vi "TorreHanoi.vi"() -> ()   [LabVIEW 2020]
uses:
  <vilib>/Utility/miscctls.llb/LVPositionTypeDef.ctl
  <vilib>/Utility/miscctls.llb/LVBoundsTypeDef.ctl
panel:
  out "String 2":string
  in  "Instrucciones":bool
  out "array1":dbl[](array[numeric])
  out "Position:Left":i32
  out "array3":dbl[](array[numeric])
  out "array2":dbl[](array[numeric])
  out "Initial position":T1
  out "CtlRef":refnum<vi>
  out "Disco4":bool caption="Disco 1"
  out "Disco3":bool caption="Disco 1"
  out "Disco5":bool caption="Disco 1"
  out "Disco2":bool caption="Disco 1"
  in  "Número de discos":u16(ring) items=["3"=3, "4"=4, "5"=5]
  out "Disco1":bool caption="Disco 1"
  out "Número de movimientos realizados":dbl
  out "Minimo de movimientos":dbl
  out "Boolean":bool
  out "Boolean 2":bool
  out "Boolean 3":bool
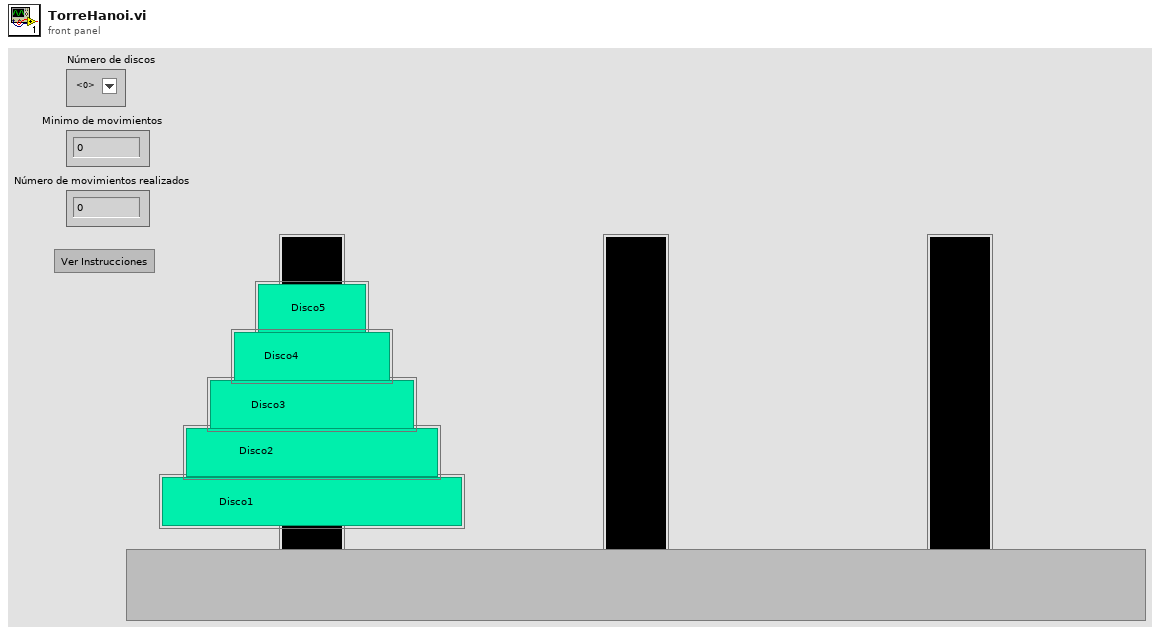
[diagram p1: front panel]
types:
  T1 = typedef "LVPositionTypeDef.ctl" = cluster{"Left":i32, "Top":i32}
  T2 = typedef "LVBoundsTypeDef.ctl" = cluster{"Width":u32, "Height":u32}
  T3 = typedef "LVPoint32TypeDef.ctl" = cluster{"Horizontal":i32, "Vertical":i32}
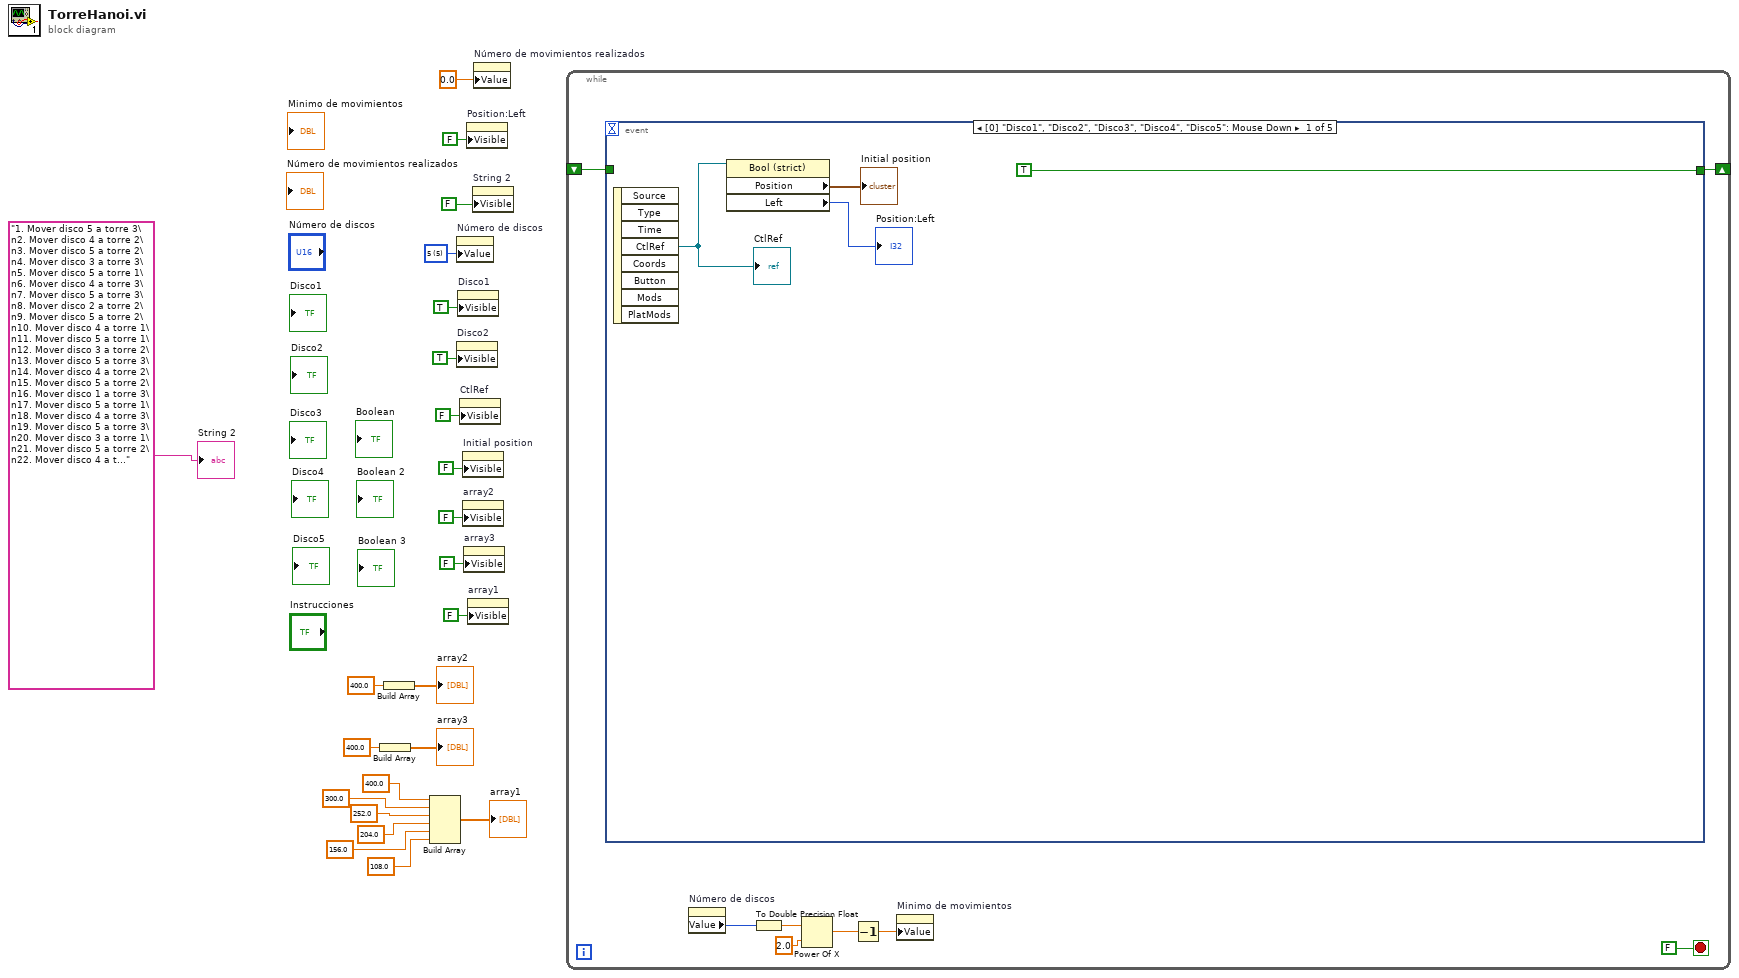
[diagram p0: block diagram]
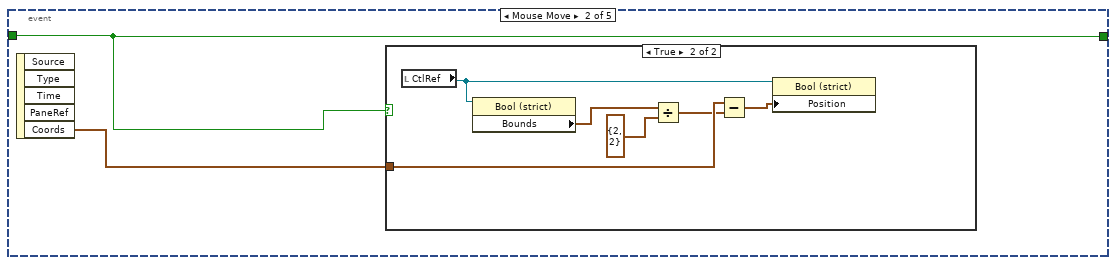
[diagram p2: hidden frame]
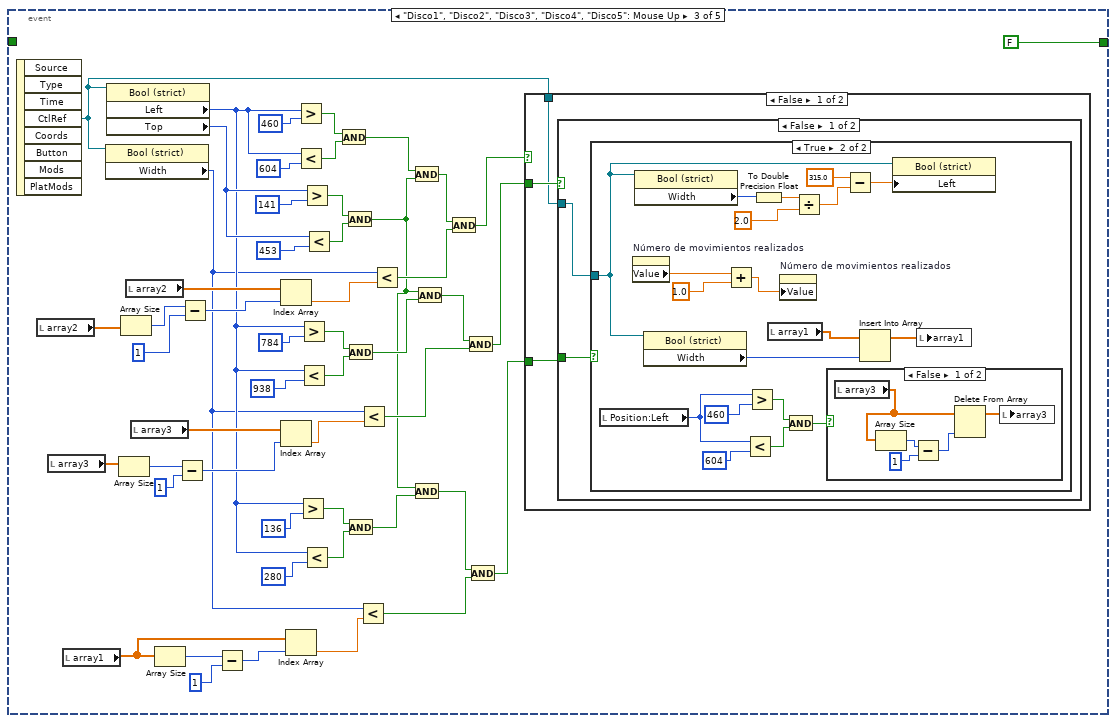
[diagram p4: hidden frame]
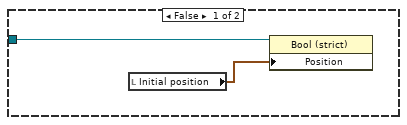
[diagram p5: hidden frame]
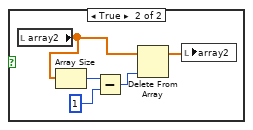
[diagram p6: hidden frame]
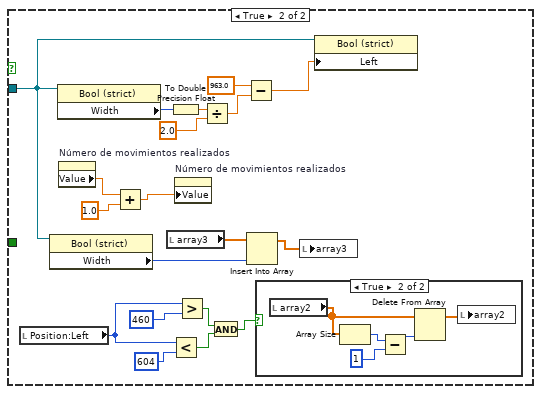
[diagram p7: hidden frame]
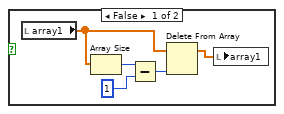
[diagram p8: hidden frame]
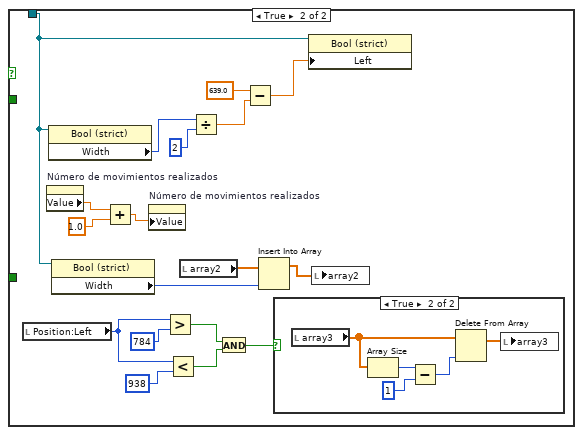
[diagram p9: hidden frame]
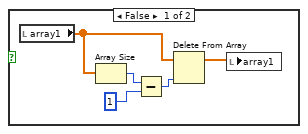
[diagram p10: hidden frame]
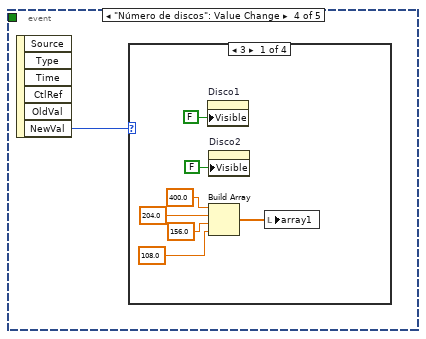
[diagram p11: hidden frame]
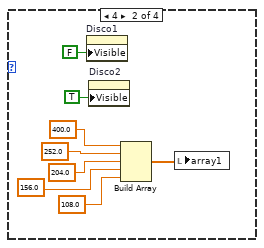
[diagram p12: hidden frame]
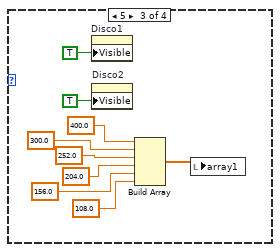
[diagram p13: hidden frame]
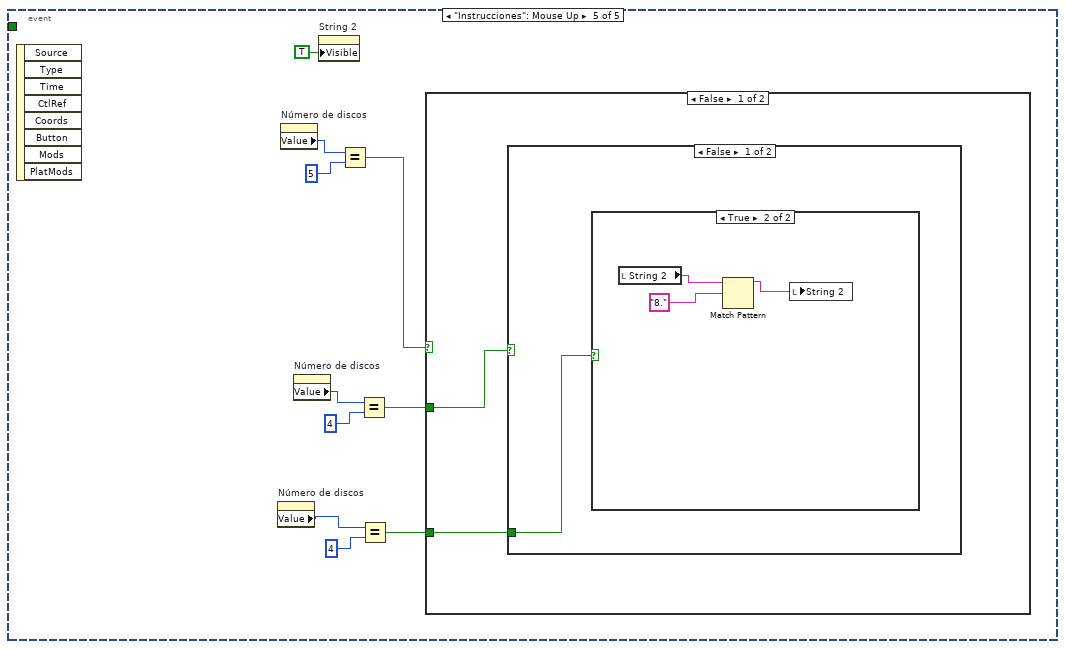
[diagram p15: hidden frame]
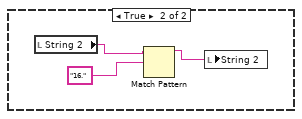
[diagram p17: hidden frame]
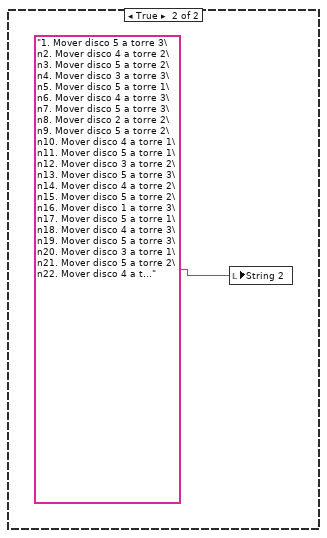
[diagram p18: hidden frame]
diagram:
  w23 = u16 5 items=["3"=3, "4"=4, "5"=5] ("Número de discos")
  n1 = Build Array(400.0 ("element")) -> (→"array3":dbl[])
  n2 = Build Array(400.0 ("element")) -> (→"array2":dbl[])
  n3 = Build Array(400.0 ("element"), 300.0 ("element"), 252.0 ("element"), 204.0 ("element"), 156.0 ("element"), 108.0 ("element")) -> (→"array1":dbl[])
  n4 = property on="Número de discos" class="Ring (strict)"("Value"=w23) -> ()  [unwired: 2 in, 2 out]
  n5 = property on="Disco2" class="Bool (strict)"("Visible"=TRUE) -> ()  [unwired: 2 in, 2 out]
  n6 = property on="Disco1" class="Bool (strict)"("Visible"=TRUE) -> ()  [unwired: 2 in, 2 out]
  n7 = property on="CtlRef" class="LVObjRef (strict)"("Visible"=FALSE) -> ()  [unwired: 2 in, 2 out]
  n8 = property on="Initial position" class="Clust (strict)"("Visible"=FALSE) -> ()  [unwired: 2 in, 2 out]
  n9 = property on="array2" class="Arr (strict)"("Visible"=FALSE) -> ()  [unwired: 2 in, 2 out]
  n10 = property on="array3" class="Arr (strict)"("Visible"=FALSE) -> ()  [unwired: 2 in, 2 out]
  n11 = property on="Position:Left" class="DigNum (strict)"("Visible"=FALSE) -> ()  [unwired: 2 in, 2 out]
  n12 = property on="array1" class="Arr (strict)"("Visible"=FALSE) -> ()  [unwired: 2 in, 2 out]
  n13 = property on="String 2" class="Str"("Visible"=FALSE) -> ()  [unwired: 2 in, 2 out]
  n14 = property on="Número de movimientos realizados" class="DigNum (strict)"("Value"=0.0 ("Número de movimientos realizados")) -> ()  [unwired: 2 in, 2 out]
  n15 = while {
    shift-right: [w25] -> _
    shift-left: _ -> [w24]
    stop <- FALSE stop-if-true
    n16 = event shown="[0] \"Disco1\", \"Disco2\", \"Disco3\", \"Disco4\", \"Disco5\": Mouse Down" {
      selector: _ -> [_ _ _ _ _]
      dyn-events: _ -> [_ _ _ _ _]
      timeout: _ -> [_ _ _ _ _]
      tunnel: [TRUE w36 FALSE _ _] -> w25
      tunnel: w24 -> [_ w36 _ _ _]
      event "Disco1", "Disco2", "Disco3", "Disco4", "Disco5": Mouse Down {
        n17 = event-data() -> ("CtlRef"=w34:refnum<vi>)  [unwired: 1 in, 7 out]
        "CtlRef" <- w34
        n18 = property class="Bool (strict)"(reference=w34) -> ("Position"=→"Initial position":T1, "Left"=→"Position:Left":i32)  [unwired: 1 in, 2 out]
      }
      event Mouse Move {
        n19 = event-data() -> ("Coords"=w37:T3)  [unwired: 1 in, 4 out]
        n20 = case shown="True" w36 {
          tunnel: w37 -> [_ w42]
          frame False {
          }
          frame True {
            n21 = local read "CtlRef"() -> (w39:refnum<vi>)
            n22 = property class="Bool (strict)"(reference=w39) -> ("Bounds"=w40:T2)  [unwired: 1 in, 2 out]
            n23 = Divide(x=w40, y=T2 {"Width"=2, "Height"=2}) -> (x/y=w41:cluster{"Width":dbl, "Height":dbl})
            n24 = Subtract(x=w42, y=w41) -> (x-y=w38:cluster{dbl, dbl})
            n25 = property class="Bool (strict)"(reference=w39, "Position"=w38) -> ()  [unwired: 1 in, 2 out]
          }
        }
      }
      event "Disco1", "Disco2", "Disco3", "Disco4", "Disco5": Mouse Up {
        n26 = event-data() -> ("CtlRef"=w78:refnum<vi>)  [unwired: 1 in, 7 out]
        n27 = local read "array2"() -> (w69:dbl[])
        n28 = local read "array3"() -> (w63:dbl[])
        n29 = local read "array1"() -> (w45:dbl[])
        n30 = property class="Bool (strict)"(reference=w78) -> ("Width"=w52:u32)  [unwired: 1 in, 2 out]
        n31 = property class="Bool (strict)"(reference=w78) -> ("Left"=w59:i32, "Top"=w83:i32)  [unwired: 1 in, 2 out]
        n32 = Array Size(array=w63) -> (size(s)=w62:i32)
        n33 = Array Size(array=w69) -> (size(s)=w67:i32)
        n34 = local read "array2"() -> (w70:dbl[])
        n35 = local read "array3"() -> (w64:dbl[])
        n36 = Array Size(array=w45) -> (size(s)=w51:i32)
        n37 = Subtract(x=w62, y=1) -> (x-y=w60:i32)
        n38 = Subtract(x=w67, y=1) -> (x-y=w68:i32)
        n39 = Subtract(x=w51, y=1) -> (x-y=w46:i32)
        n40 = Index Array(array=w70, index=w68) -> (element=w71:dbl)
        n41 = Index Array(array=w64, index=w60) -> (element=w65:dbl)
        n42 = Index Array(array=w45, index=w46) -> (element=w44:dbl)
        n43 = Greater?(x=w59, y=460) -> (0:w91:bool)
        n44 = Less?(x=w59, y=604) -> (x < y?=w90:bool)
        n45 = Greater?(x=w59, y=136) -> (0:w56:bool)
        n46 = Greater?(x=w59, y=784) -> (0:w89:bool)
        n47 = Less?(x=w59, y=938) -> (x < y?=w88:bool)
        n48 = Greater?(x=w83, y=141) -> (0:w85:bool)
        n49 = Less?(x=w59, y=280) -> (x < y?=w55:bool)
        n50 = Less?(x=w83, y=453) -> (x < y?=w84:bool)
        n51 = And(x=w91, y=w90) -> (x .and. y?=w80:bool)
        n52 = And(x=w85, y=w84) -> (x .and. y?=w54:bool)
        n53 = And(x=w89, y=w88) -> (x .and. y?=w79:bool)
        n54 = And(x=w56, y=w55) -> (x .and. y?=w53:bool)
        n55 = Less?(x=w52, y=w44) -> (x < y?=w49:bool)
        n56 = Less?(x=w52, y=w65) -> (x < y?=w74:bool)
        n57 = Less?(x=w52, y=w71) -> (x < y?=w77:bool)
        n58 = And(x=w80, y=w54) -> (x .and. y?=w76:bool)
        n59 = And(x=w54, y=w53) -> (x .and. y?=w48:bool)
        n60 = And(x=w54, y=w79) -> (x .and. y?=w73:bool)
        n61 = And(x=w76, y=w77) -> (x .and. y?=w75:bool)
        n62 = And(x=w73, y=w74) -> (x .and. y?=w72:bool)
        n63 = And(x=w48, y=w49) -> (x .and. y?=w47:bool)
        n64 = case shown="False" w75 {
          tunnel: w78 -> [w96 w169]
          tunnel: w72 -> [w97 _]
          tunnel: w47 -> [w95 _]
          frame False {
            n65 = case shown="False" w97 {
              tunnel: w96 -> [w99 w143]
              tunnel: w95 -> [w98 _]
              frame False {
                n66 = case shown="True" w98 {
                  tunnel: w99 -> [w100 w111]
                  frame False {
                    n67 = local read "Initial position"() -> (w101:T1)
                    n68 = property class="Bool (strict)"(reference=w100, "Position"=w101) -> ()  [unwired: 1 in, 2 out]
                  }
                  frame True {
                    n69 = local read "Position:Left"() -> (w107:i32)
                    n70 = property on="Número de movimientos realizados" class="DigNum (strict)"() -> ("Value"=w114:dbl)  [unwired: 2 in, 2 out]
                    n71 = property class="Bool (strict)"(reference=w111) -> ("Width"=w120:u32)  [unwired: 1 in, 2 out]
                    n72 = property class="Bool (strict)"(reference=w111) -> ("Width"=w110:u32)  [unwired: 1 in, 2 out]
                    n73 = Add(x=w114, y=1.0) -> (x+y=w112:dbl)
                    n74 = Less?(x=w107, y=604) -> (x < y?=w103:bool)
                    n75 = Greater?(x=w107, y=460) -> (0:w104:bool)
                    n76 = To Double Precision Float(number=w120) -> (double precision float=w119:dbl)
                    n77 = local read "array1"() -> (w109:dbl[])
                    n78 = property on="Número de movimientos realizados" class="DigNum (strict)"("Value"=w112) -> ()  [unwired: 2 in, 2 out]
                    n79 = And(x=w104, y=w103) -> (x .and. y?=w102:bool)
                    n80 = Divide(x=w119, y=2.0) -> (x/y=w117:dbl)
                    n81 = case shown="False" w102 {
                      frame False {
                        n82 = local read "array3"() -> (w124:dbl[])
                        n83 = Array Size(array=w124) -> (size(s)=w123:i32)
                        n84 = Subtract(x=w123, y=1) -> (x-y=w121:i32)
                        n85 = Delete From Array(array=w124, index=w121) -> (array with subset deleted=w125:dbl[])  [unwired: 1 in, 1 out]
                        n86 = local write "array3"(w125) -> ()
                      }
                      frame True {
                        n87 = local read "array2"() -> (w129:dbl[])
                        n88 = Array Size(array=w129) -> (size(s)=w128:i32)
                        n89 = Subtract(x=w128, y=1) -> (x-y=w126:i32)
                        n90 = Delete From Array(array=w129, index=w126) -> (array with subset deleted=w130:dbl[])  [unwired: 1 in, 1 out]
                        n91 = local write "array2"(w130) -> ()
                      }
                    }
                    n92 = Subtract(x=315.0, y=w117) -> (x-y=w115:dbl)
                    n93 = Insert Into Array(array=w109, new element=w110) -> (w108:dbl[])  [unwired: 1 in]
                    n94 = property class="Bool (strict)"(reference=w111, "Left"=w115) -> ()  [unwired: 1 in, 2 out]
                    n95 = local write "array1"(w108) -> ()
                  }
                }
              }
              frame True {
                n96 = local read "Position:Left"() -> (w137:i32)
                n97 = property class="Bool (strict)"(reference=w143) -> ("Width"=w140:u32)  [unwired: 1 in, 2 out]
                n98 = property class="Bool (strict)"(reference=w143) -> ("Width"=w142:u32)  [unwired: 1 in, 2 out]
                n99 = property on="Número de movimientos realizados" class="DigNum (strict)"() -> ("Value"=w146:dbl)  [unwired: 2 in, 2 out]
                n100 = Add(x=w146, y=1.0) -> (x+y=w144:dbl)
                n101 = local read "array3"() -> (w139:dbl[])
                n102 = To Double Precision Float(number=w142) -> (double precision float=w141:dbl)
                n103 = Less?(x=w137, y=604) -> (x < y?=w133:bool)
                n104 = property on="Número de movimientos realizados" class="DigNum (strict)"("Value"=w144) -> ()  [unwired: 2 in, 2 out]
                n105 = Greater?(x=w137, y=460) -> (0:w134:bool)
                n106 = Divide(x=w141, y=2.0) -> (x/y=w149:dbl)
                n107 = And(x=w134, y=w133) -> (x .and. y?=w132:bool)
                n108 = Subtract(x=963.0, y=w149) -> (x-y=w147:dbl)
                n109 = Insert Into Array(array=w139, new element=w140) -> (w138:dbl[])  [unwired: 1 in]
                n110 = case shown="True" w132 {
                  frame False {
                    n111 = local read "array1"() -> (w153:dbl[])
                    n112 = Array Size(array=w153) -> (size(s)=w151:i32)
                    n113 = Subtract(x=w151, y=1) -> (x-y=w152:i32)
                    n114 = Delete From Array(array=w153, index=w152) -> (array with subset deleted=w154:dbl[])  [unwired: 1 in, 1 out]
                    n115 = local write "array1"(w154) -> ()
                  }
                  frame True {
                    n116 = local read "array2"() -> (w159:dbl[])
                    n117 = Array Size(array=w159) -> (size(s)=w157:i32)
                    n118 = Subtract(x=w157, y=1) -> (x-y=w158:i32)
                    n119 = Delete From Array(array=w159, index=w158) -> (array with subset deleted=w155:dbl[])  [unwired: 1 in, 1 out]
                    n120 = local write "array2"(w155) -> ()
                  }
                }
                n121 = local write "array3"(w138) -> ()
                n122 = property class="Bool (strict)"(reference=w143, "Left"=w147) -> ()  [unwired: 1 in, 2 out]
              }
            }
          }
          frame True {
            n123 = local read "Position:Left"() -> (w165:i32)
            n124 = property on="Número de movimientos realizados" class="DigNum (strict)"() -> ("Value"=w171:dbl)  [unwired: 2 in, 2 out]
            n125 = property class="Bool (strict)"(reference=w169) -> ("Width"=w176:u32)  [unwired: 1 in, 2 out]
            n126 = property class="Bool (strict)"(reference=w169) -> ("Width"=w168:u32)  [unwired: 1 in, 2 out]
            n127 = Add(x=w171, y=1.0 ("x")) -> (x+y=w172:dbl)
            n128 = property on="Número de movimientos realizados" class="DigNum (strict)"("Value"=w172) -> ()  [unwired: 2 in, 2 out]
            n129 = Greater?(x=w165, y=784) -> (0:w162:bool)
            n130 = Less?(x=w165, y=938) -> (x < y?=w161:bool)
            n131 = local read "array2"() -> (w167:dbl[])
            n132 = Divide(x=w176, y=u32 2) -> (x/y=w174:dbl)
            n133 = And(x=w162, y=w161) -> (x .and. y?=w160:bool)
            n134 = Subtract(x=639.0, y=w174) -> (x-y=w173:dbl)
            n135 = Insert Into Array(array=w167, new element=w168) -> (w166:dbl[])  [unwired: 1 in]
            n136 = case shown="True" w160 {
              frame False {
                n137 = local read "array1"() -> (w181:dbl[])
                n138 = Array Size(array=w181) -> (size(s)=w179:i32)
                n139 = Subtract(x=w179, y=1) -> (x-y=w180:i32)
                n140 = Delete From Array(array=w181, index=w180) -> (array with subset deleted=w182:dbl[])  [unwired: 1 in, 1 out]
                n141 = local write "array1"(w182) -> ()
              }
              frame True {
                n142 = local read "array3"() -> (w187:dbl[])
                n143 = Array Size(array=w187) -> (size(s)=w185:i32)
                n144 = Subtract(x=w185, y=1) -> (x-y=w183:i32)
                n145 = Delete From Array(array=w187, index=w183) -> (array with subset deleted=w186:dbl[])  [unwired: 1 in, 1 out]
                n146 = local write "array3"(w186) -> ()
              }
            }
            n147 = property class="Bool (strict)"(reference=w169, "Left"=w173) -> ()  [unwired: 1 in, 2 out]
            n148 = local write "array2"(w166) -> ()
          }
        }
      }
      event "Número de discos": Value Change {
        n149 = event-data() -> ("NewVal"=w188:u16)  [unwired: 1 in, 5 out]
        n150 = case shown="3" w188 {
          frame 3 {
            n151 = property on="Disco1" class="Bool (strict)"("Visible"=FALSE) -> ()  [unwired: 2 in, 2 out]
            n152 = property on="Disco2" class="Bool (strict)"("Visible"=FALSE) -> ()  [unwired: 2 in, 2 out]
            n153 = Build Array(400.0 ("element"), 204.0 ("element"), 156.0 ("element"), 108.0 ("element")) -> (w189:dbl[])
            n154 = local write "array1"(w189) -> ()
          }
          frame 4 {
            n155 = property on="Disco1" class="Bool (strict)"("Visible"=FALSE) -> ()  [unwired: 2 in, 2 out]
            n156 = property on="Disco2" class="Bool (strict)"("Visible"=TRUE) -> ()  [unwired: 2 in, 2 out]
            n157 = Build Array(400.0 ("element"), 252.0 ("element"), 204.0 ("element"), 156.0 ("element"), 108.0 ("element")) -> (w196:dbl[])
            n158 = local write "array1"(w196) -> ()
          }
          frame 5 {
            n159 = property on="Disco1" class="Bool (strict)"("Visible"=TRUE) -> ()  [unwired: 2 in, 2 out]
            n160 = property on="Disco2" class="Bool (strict)"("Visible"=TRUE) -> ()  [unwired: 2 in, 2 out]
            n161 = Build Array(400.0 ("element"), 300.0 ("element"), 252.0 ("element"), 204.0 ("element"), 156.0 ("element"), 108.0 ("element")) -> (w207:dbl[])
            n162 = local write "array1"(w207) -> ()
          }
          frame Default {
          }
        }
      }
      event "Instrucciones": Mouse Up {
        n163 = event-data() -> ()  [unwired: 1 in, 8 out]
        n164 = property on="Número de discos" class="Ring (strict)"() -> ("Value"=w214:u16)  [unwired: 2 in, 2 out]
        n165 = property on="Número de discos" class="Ring (strict)"() -> ("Value"=w221:u16)  [unwired: 2 in, 2 out]
        n166 = property on="Número de discos" class="Ring (strict)"() -> ("Value"=w217:u16)  [unwired: 2 in, 2 out]
        n167 = property on="String 2" class="Str"("Visible"=TRUE) -> ()  [unwired: 2 in, 2 out]
        n168 = Equal?(x=w221, y=u16 5) -> (x = y?=w219:bool)
        n169 = Equal?(x=w217, y=u16 4) -> (x = y?=w216:bool)
        n170 = Equal?(x=w214, y=u16 4) -> (x = y?=w213:bool)
        n171 = case shown="False" w219 {
          tunnel: w216 -> [w224 _]
          tunnel: w213 -> [w223 _]
          frame False {
            n172 = case shown="False" w224 {
              tunnel: w223 -> [w225 _]
              frame False {
                n173 = case shown="True" w225 {
                  frame False {
                  }
                  frame True {
                    n174 = local read "String 2"() -> (w228:string)
                    n175 = Match Pattern(string=w228, regular expression="8.") -> (before substring=w226:string)  [unwired: 1 in, 3 out]
                    n176 = local write "String 2"(w226) -> ()
                  }
                }
              }
              frame True {
                n177 = local read "String 2"() -> (w231:string)
                n178 = Match Pattern(string=w231, regular expression="16.") -> (before substring=w229:string)  [unwired: 1 in, 3 out]
                n179 = local write "String 2"(w229) -> ()
              }
            }
          }
          frame True {
            n180 = local write "String 2"("1. Mover disco 5 a torre 3\n2. Mover disco 4 a torre 2\n3. Mover disco 5 a torre 2\n4. Mover disco 3 a torre 3\n5. Mover disco 5 a torre 1\n6. Mover disco 4 a torre 3\n7. Mover disco 5 a torre 3\n8. Mover disco 2 a torre 2\n9. Mover disco 5 a torre 2\n10. Mover disco 4 a torre 1\n11. Mover disco 5 a torre 1\n12. Mover disco 3 a torre 2\n13. Mover disco 5 a torre 3\n14. Mover disco 4 a torre 2\n15. Mover disco 5 a torre 2\n16. Mover disco 1 a torre 3\n17. Mover disco 5 a torre 1\n18. Mover disco 4 a torre 3\n19. Mover disco 5 a torre 3\n20. Mover disco 3 a torre 1\n21. Mover disco 5 a torre 2\n22. Mover disco 4 a torre 1\n23. Mover disco 5 a torre 1\n24. Mover disco 2 a torre 3\n25. Mover disco 5 a torre 3\n26. Mover disco 4 a torre 2\n27. Mover disco 5 a torre 2\n28. Mover disco 3 a torre 3\n29. Mover disco 5 a torre 1\n30. Mover disco 2 a torre 3\n31. Mover disco 1 a torre 3" ("String")) -> ()
          }
        }
      }
    }
    n181 = property on="Número de discos" class="Ring (strict)"() -> ("Value"=w26:u16)  [unwired: 2 in, 2 out]
    n182 = To Double Precision Float(number=w26) -> (double precision float=w29:dbl)
    n183 = Power Of X(1:2.0 ("x"), 2:w29) -> (0:w30:dbl)
    n184 = Decrement(x=w30) -> (x-1=w27:dbl)
    n185 = property on="Minimo de movimientos" class="DigNum (strict)"("Value"=w27) -> ()  [unwired: 2 in, 2 out]
  }
  "String 2" <- "1. Mover disco 5 a torre 3\n2. Mover disco 4 a torre 2\n3. Mover disco 5 a torre 2\n4. Mover disco 3 a torre 3\n5. Mover disco 5 a torre 1\n6. Mover disco 4 a torre 3\n7. Mover disco 5 a torre 3\n8. Mover disco 2 a torre 2\n9. Mover disco 5 a torre 2\n10. Mover disco 4 a torre 1\n11. Mover disco 5 a torre 1\n12. Mover disco 3 a torre 2\n13. Mover disco 5 a torre 3\n14. Mover disco 4 a torre 2\n15. Mover disco 5 a torre 2\n16. Mover disco 1 a torre 3\n17. Mover disco 5 a torre 1\n18. Mover disco 4 a torre 3\n19. Mover disco 5 a torre 3\n20. Mover disco 3 a torre 1\n21. Mover disco 5 a torre 2\n22. Mover disco 4 a torre 1\n23. Mover disco 5 a torre 1\n24. Mover disco 2 a torre 3\n25. Mover disco 5 a torre 3\n26. Mover disco 4 a torre 2\n27. Mover disco 5 a torre 2\n28. Mover disco 3 a torre 3\n29. Mover disco 5 a torre 1\n30. Mover disco 2 a torre 3\n31. Mover disco 1 a torre 3" ("String")
